vi "Convert to scripting configuration.vi"(7 "GObj Array in":refnum<vi>[](array[refnum]), 8 "error in (no error)":errorcluster, 11 "Multiple Assert Configuration":T1[](array[typedef])) -> (0 "error out":errorcluster, 3 "Array":T4[](array[typedef]), 5 "GObj Array out":refnum<vi>[](array[refnum]))   [LabVIEW 2016]
doc: "Converts the simplified multiple assert configuration array into the full scripting configuration"
uses:
  Assert Scripting Configuration.ctl
  <vilib>/Utility/Data Type/Type Definitions/Data Type.ctl
  Assert Build Configuration.ctl
  Core/Assert API Components/Failure Actions.ctl
  <vilib>/Utility/Data Type/NI_Data Type.lvlib
  Core/Assert API Components/Assert API Components.lvlib
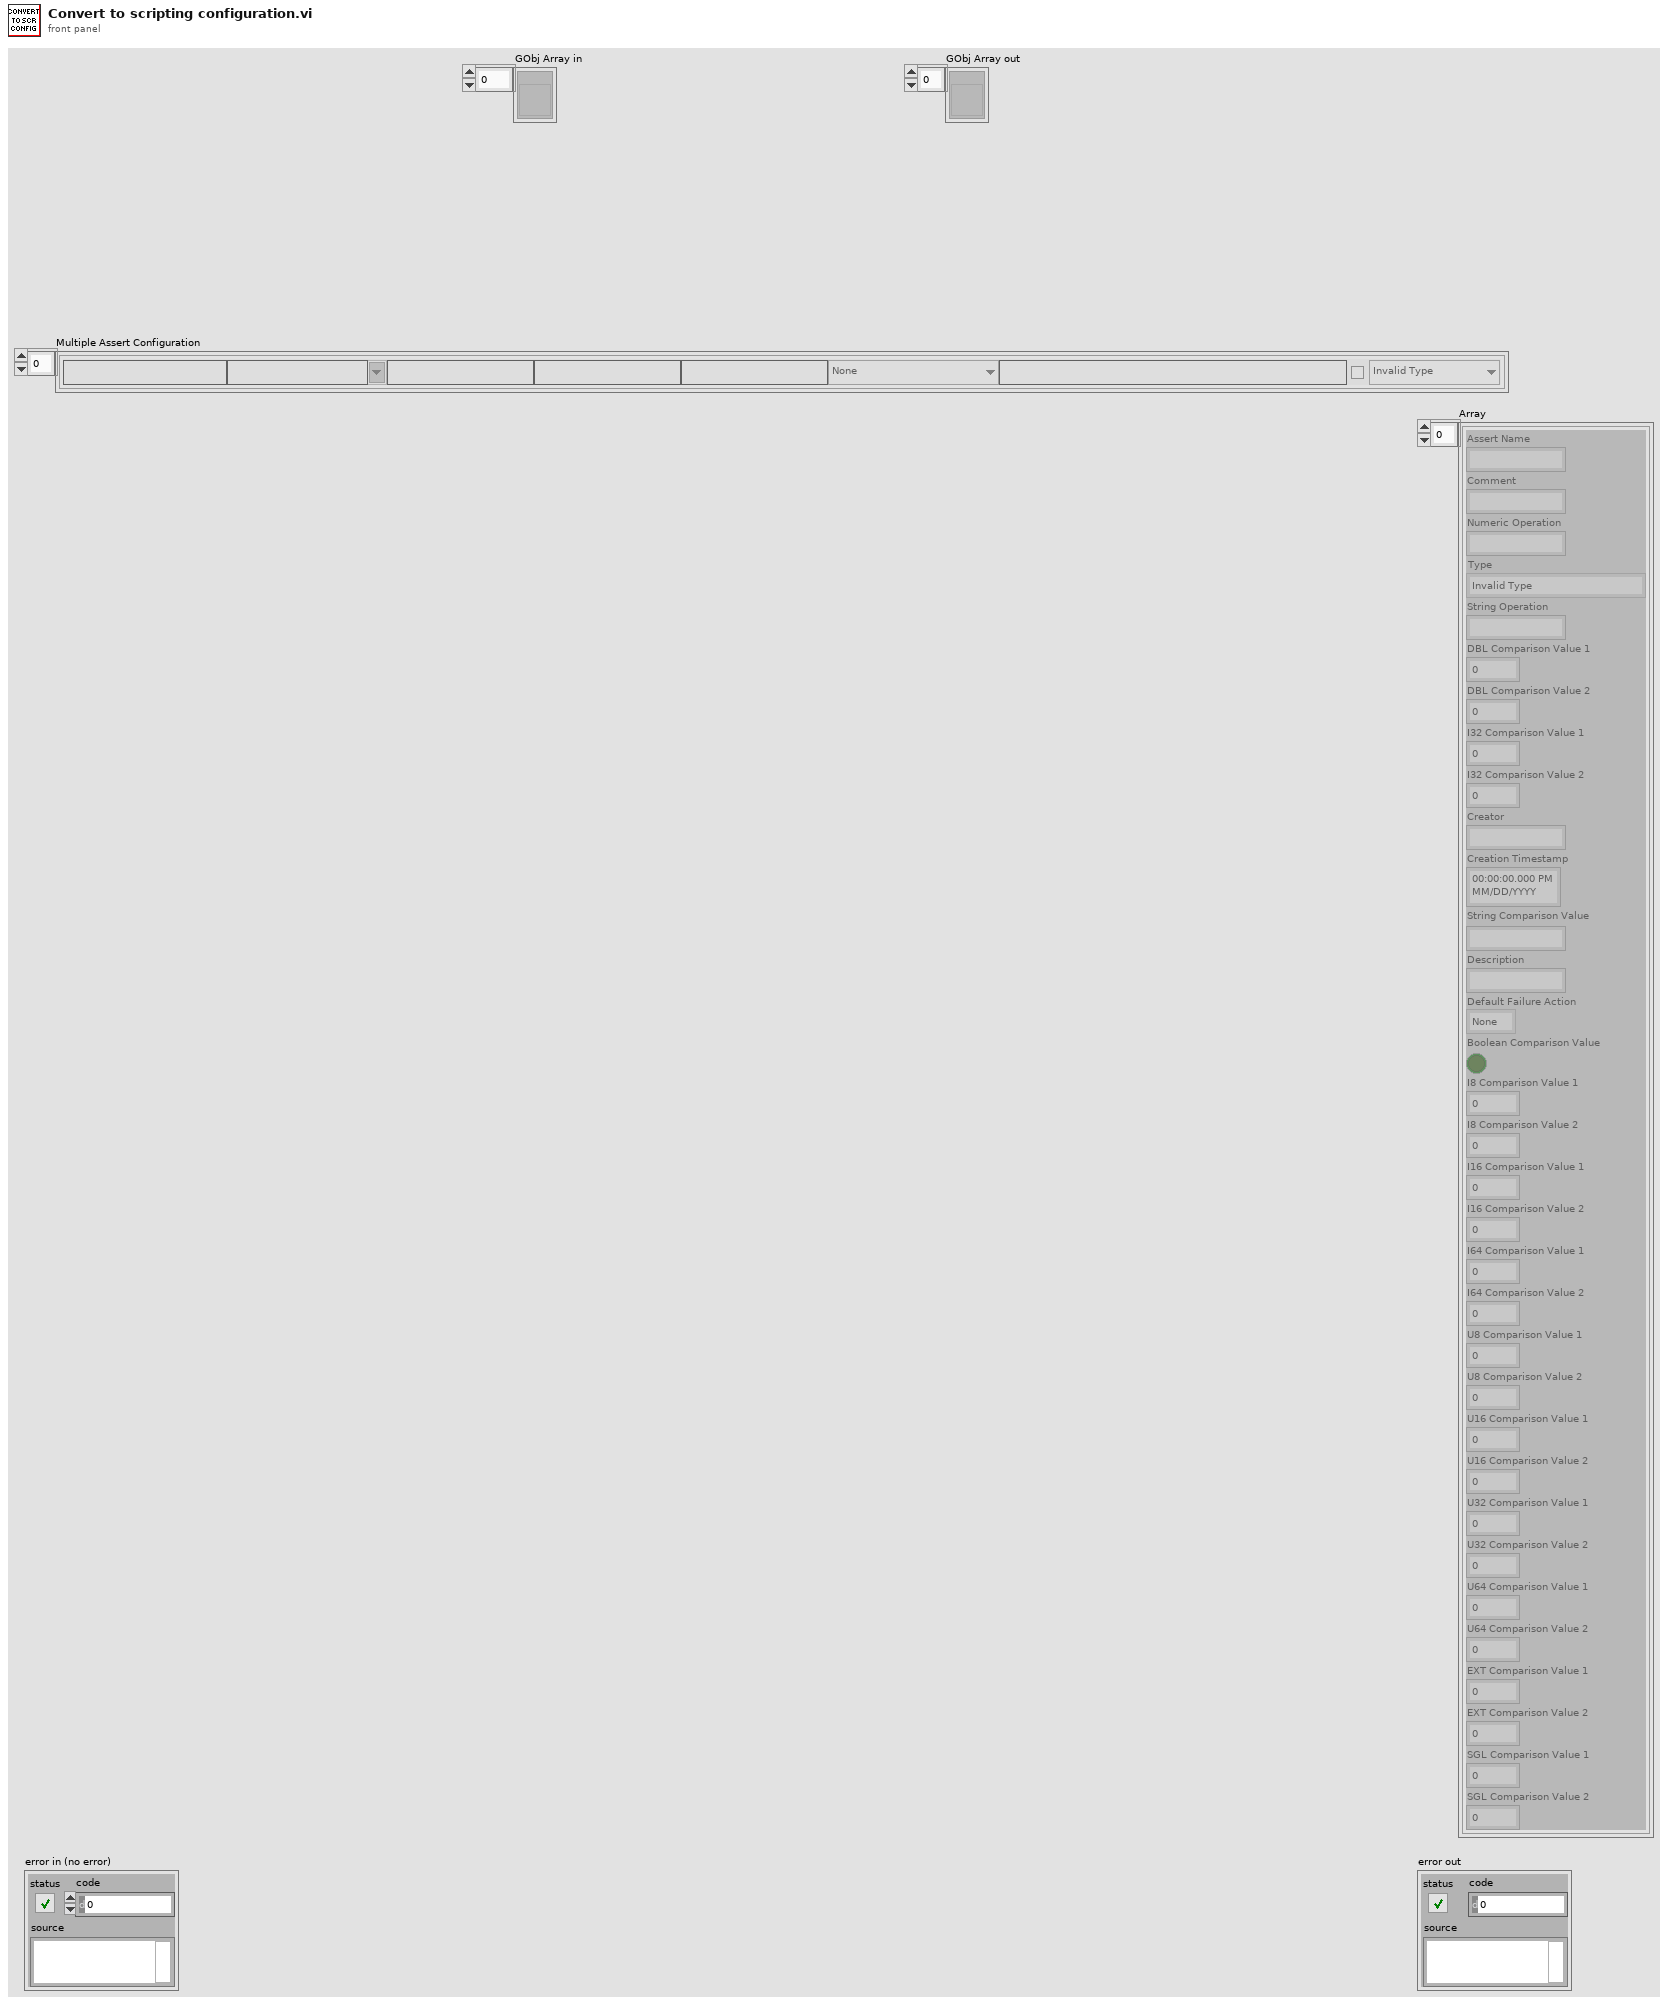
[diagram p1: front panel]
types:
  T1 = typedef "Assert Build Configuration.ctl" = cluster{"Assert Name":string, "Operation":string, "Comparison Value 1":string, "Comparison Value 2":string, "Comment":string, "Default Failure Action":T2, "Description":string, "Operation Display":string, "Active":bool, "Data Type":T3}
  T2 = typedef "Assert API Components.lvlib/Failure Actions.ctl" = enum16{"None", "Log To File", "Pause Execution", "Abort Execution"}
  T3 = typedef "NI_Data Type.lvlib/Data Type.ctl" = enum8{"Invalid Type", "Void", "I8", "I16", "I32", "I64", "U8", "U16", "U32", "U64", "Single Float", "Double Float", "Extended Float", "Single Complex", "Double Complex", "Extended Complex", "Enum U8", "Enum U16", "Enum U32", "Enum U64", "Single Float With Unit", "Double Float With Unit", "Extended Float With Unit", "Single Complex with Unit", "Double Complex with Unit", "Extended Complex with Unit", "Boolean", "String", "Path", "Picture", "Tag", "Array", "Cluster", "Variant", "LV Variant", "Waveform", "Timestamp", "Digital Waveform", "Digital Data", "ExpressData", "Refnum", "External Data", "VI", "Poly VI", "LabVIEW Class Instance", "Fixed Point"}
  T4 = typedef "Assert Scripting Configuration.ctl" = cluster{"Assert Name":string, "Comment":string, "Numeric Operation":string, "Type":T3, "String Operation":string, "DBL Comparison Value 1":dbl, "DBL Comparison Value 2":dbl, "I32 Comparison Value 1":i32, "I32 Comparison Value 2":i32, "Creator":string, "Creation Timestamp":timestamp, "String Comparison Value":string, "Description":string, "Default Failure Action":enum16{"None", "Log To File", "Pause Execution", "Abort Execution"}, "Boolean Comparison Value":bool, "I8 Comparison Value 1":i8, "I8 Comparison Value 2":i8, "I16 Comparison Value 1":i16, "I16 Comparison Value 2":i16, "I64 Comparison Value 1":i64, "I64 Comparison Value 2":i64, "U8 Comparison Value 1":u8, "U8 Comparison Value 2":u8, "U16 Comparison Value 1":u16, "U16 Comparison Value 2":u16, "U32 Comparison Value 1":u32, "U32 Comparison Value 2":u32, "U64 Comparison Value 1":u64, "U64 Comparison Value 2":u64, "EXT Comparison Value 1":ext, "EXT Comparison Value 2":ext, "SGL Comparison Value 1":sgl, "SGL Comparison Value 2":sgl}
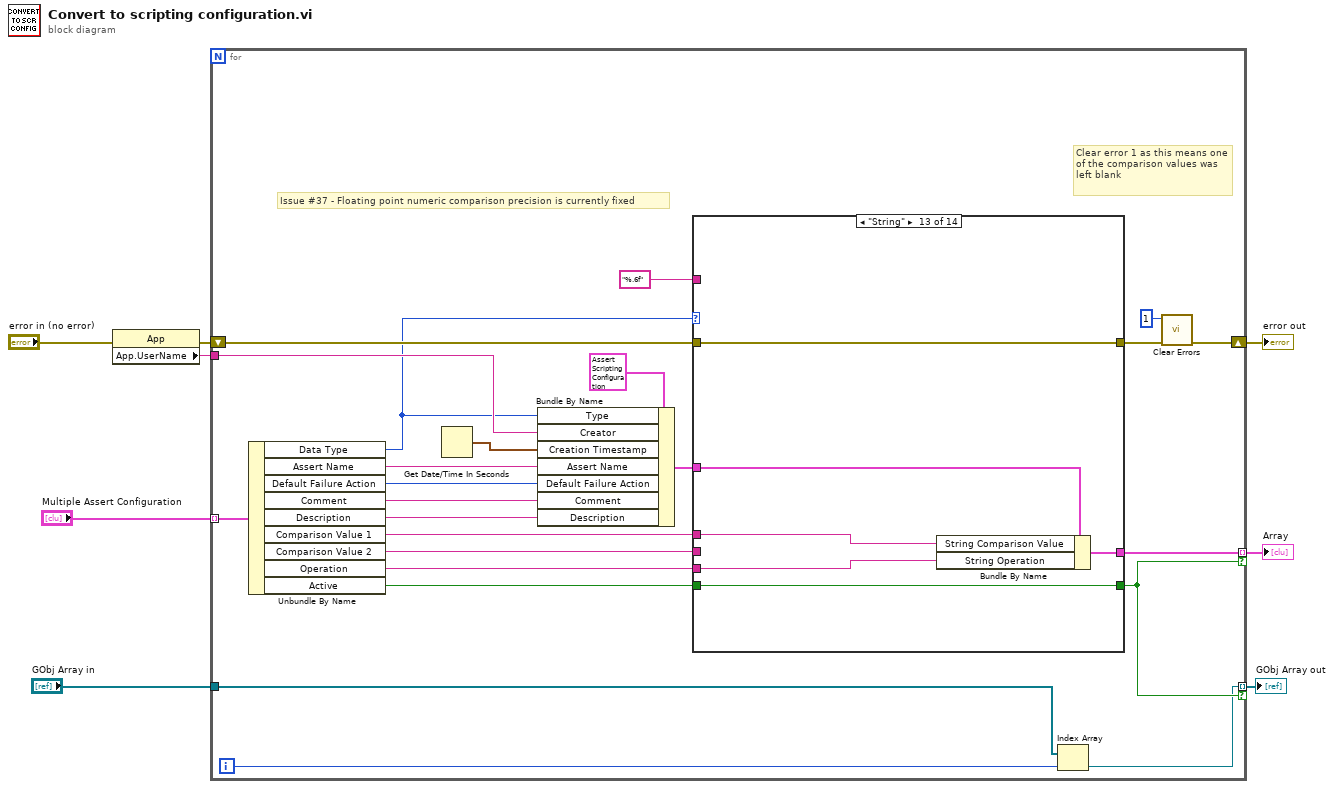
[diagram p0: block diagram]
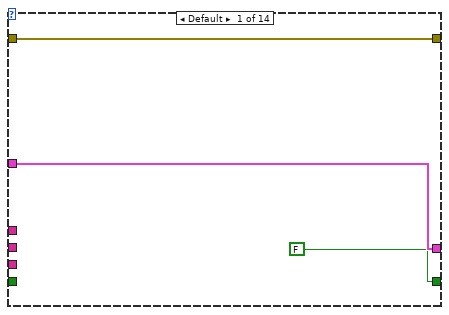
[diagram p2: hidden frame]
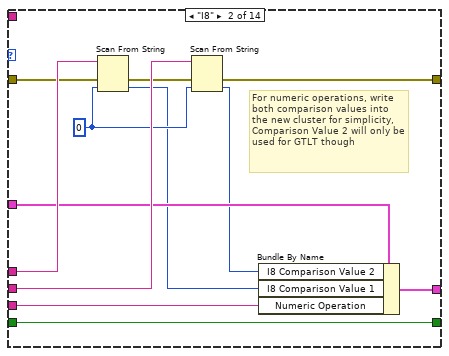
[diagram p3: hidden frame]
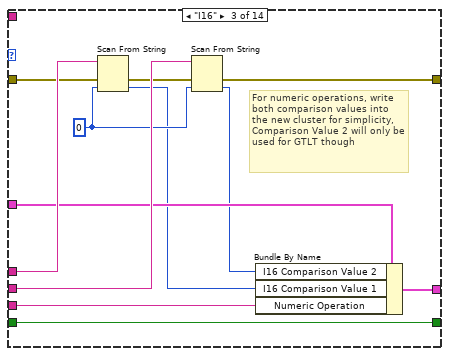
[diagram p4: hidden frame]
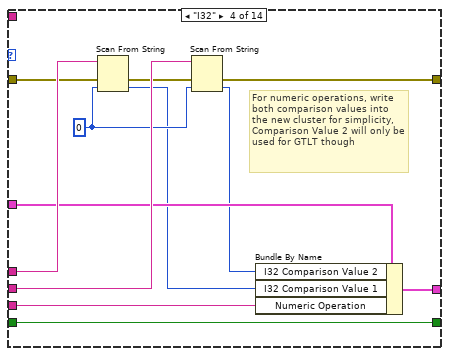
[diagram p5: hidden frame]
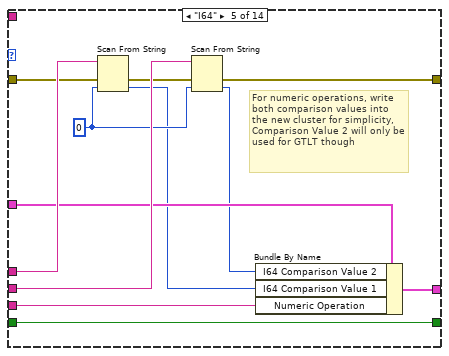
[diagram p6: hidden frame]
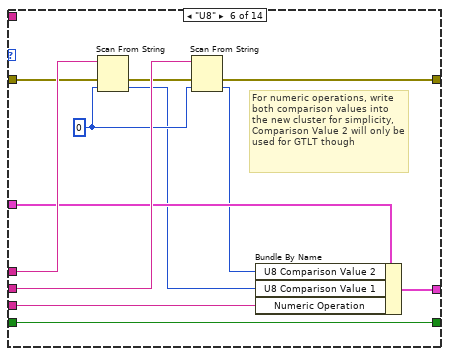
[diagram p7: hidden frame]
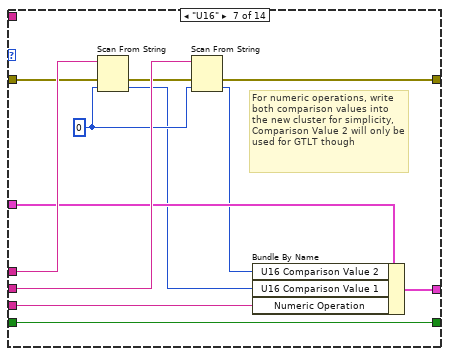
[diagram p8: hidden frame]
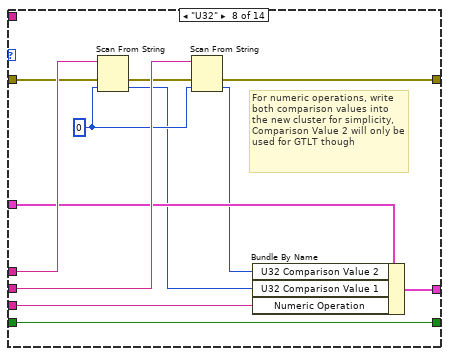
[diagram p9: hidden frame]
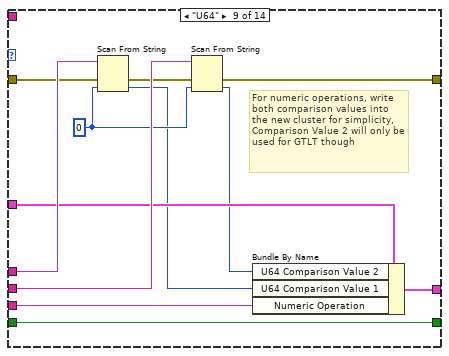
[diagram p10: hidden frame]
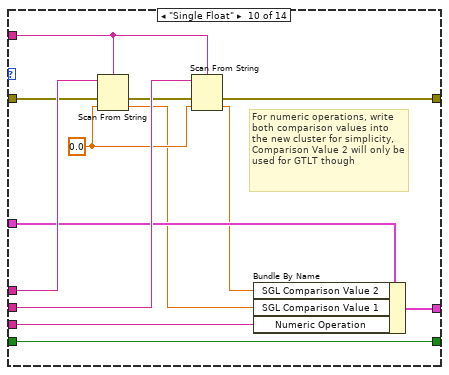
[diagram p11: hidden frame]
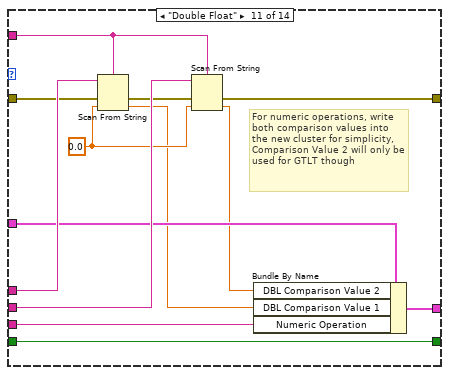
[diagram p12: hidden frame]
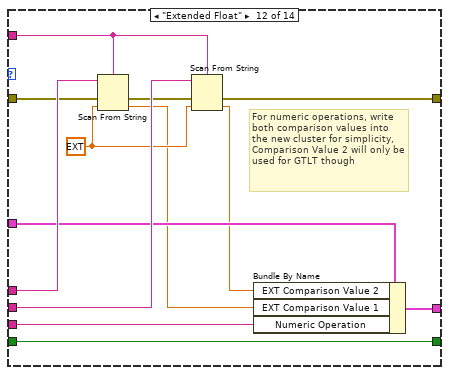
[diagram p13: hidden frame]
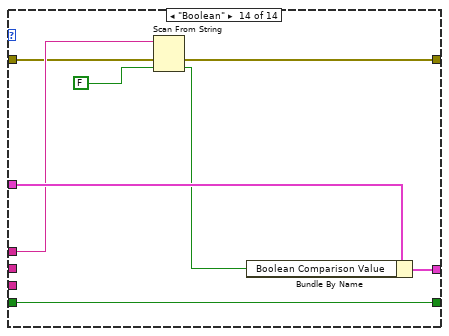
[diagram p14: hidden frame]
diagram:
  n1 = property class="App"(error in="error in (no error)") -> (error out=w5:errorcluster, "App.UserName"=w6:string)  [unwired: 1 in, 1 out]
  n2 = for {
    tunnel: "Multiple Assert Configuration" -> [w32] mode=indexing
    tunnel: w6 -> [w26]
    tunnel: [w23] -> w3 mode=indexing if=w12
    shift-right: [w15] -> w4
    shift-left: w5 -> [w19]
    tunnel: "GObj Array in" -> [w11]
    tunnel: [w9] -> w1 mode=indexing if=w12
    i -> [w10]
    # "Issue #37 - Floating point numeric comparison precision is currently fixed"
    # "Clear error 1 as this means one of the comparison values was left blank"
    n3 = Unbundle By Name(w32) -> ("Data Type"=w16:T3, "Assert Name"=w31:string, "Default Failure Action"=w30:T2, "Comment"=w29:string, "Description"=w28:string, "Comparison Value 1"=w20:string, "Comparison Value 2"=w21:string, "Operation"=w22:string, "Active"=w24:bool)
    n4 = Get Date/Time In Seconds() -> (seconds since 1Jan1904=w27:timestamp)
    n5 = Bundle By Name(cluster=T4 {"Assert Name"="", "Comment"="", "Numeric Operation"="", "Type"=enum."Double Float", "String Operation"="", "DBL Comparison Value 1"=0.0, "DBL Comparison Value 2"=0.0, "I32 Comparison Value 1"=0, "I32 Comparison Value 2"=0, "Creator"="", "Creation Timestamp"=timestamp(0 s since 1904-01-01), "String Comparison Value"="", "Description"="", "Default Failure Action"=enum."None", "Boolean Comparison Value"=FALSE, "I8 Comparison Value 1"=0, "I8 Comparison Value 2"=0, "I16 Comparison Value 1"=0, "I16 Comparison Value 2"=0, "I64 Comparison Value 1"=0, "I64 Comparison Value 2"=0, "U8 Comparison Value 1"=0, "U8 Comparison Value 2"=0, "U16 Comparison Value 1"=0, "U16 Comparison Value 2"=0, "U32 Comparison Value 1"=0, "U32 Comparison Value 2"=0, "U64 Comparison Value 1"=0, "U64 Comparison Value 2"=0, "EXT Comparison Value 1"=0.0, "EXT Comparison Value 2"=0.0, "SGL Comparison Value 1"=0.0, "SGL Comparison Value 2"=0.0} ("Assert Scripting Configuration"), "Type"=w16, "Creator"=w26, "Creation Timestamp"=w27, "Assert Name"=w31, "Default Failure Action"=w30, "Comment"=w29, "Description"=w28) -> (w25:T4)
    n6 = case shown="\"String\"" w16 {
      tunnel: w25 -> [w35 w44 w56 w68 w80 w92 w104 w116 w128 w141 w154 w167 w175 w183]
      tunnel: w24 -> [_ w45 w57 w69 w81 w93 w105 w117 w129 w142 w155 w168 w176 w184]
      tunnel: [w35 w42 w54 w66 w78 w90 w102 w114 w126 w139 w152 w165 w173 w182] -> w23
      tunnel: [FALSE w45 w57 w69 w81 w93 w105 w117 w129 w142 w155 w168 w176 w184] -> w12
      tunnel: w22 -> [_ w38 w50 w62 w74 w86 w98 w110 w122 w135 w148 w161 w172 _]
      tunnel: w21 -> [_ w47 w59 w71 w83 w95 w107 w119 w131 w144 w157 w170 _ _]
      tunnel: w20 -> [_ w46 w58 w70 w82 w94 w106 w118 w130 w143 w156 w169 w171 w181]
      tunnel: w19 -> [w33 w43 w55 w67 w79 w91 w103 w115 w127 w140 w153 w166 w174 w178]
      tunnel: [w33 w41 w53 w65 w77 w89 w101 w113 w125 w138 w151 w164 w174 w177] -> w18
      tunnel: "%.6f" ("format string") -> [_ _ _ _ _ _ _ _ _ w132 w145 w158 _ _]
      frame Default {
      }
      frame "I8" {
        w39 = i8 0
        # "For numeric operations, write both comparison values into the new cluster for simplicity, Comparison Value 2 will only be used for GTLT though"
        n7 = Scan From String(input string=w46, error in=w43, default 1=w39) -> (error out=w40:errorcluster, output 1=w36:i8)  [unwired: 2 in, 2 out]
        n8 = Scan From String(input string=w47, error in=w40, default 1=w39) -> (error out=w41:errorcluster, output 1=w37:i8)  [unwired: 2 in, 2 out]
        n9 = Bundle By Name(cluster=w44, "I8 Comparison Value 2"=w37, "I8 Comparison Value 1"=w36, "Numeric Operation"=w38) -> (w42:T4)
      }
      frame "I16" {
        w51 = i16 0
        # "For numeric operations, write both comparison values into the new cluster for simplicity, Comparison Value 2 will only be used for GTLT though"
        n10 = Scan From String(input string=w58, error in=w55, default 1=w51) -> (error out=w52:errorcluster, output 1=w48:i16)  [unwired: 2 in, 2 out]
        n11 = Scan From String(input string=w59, error in=w52, default 1=w51) -> (error out=w53:errorcluster, output 1=w49:i16)  [unwired: 2 in, 2 out]
        n12 = Bundle By Name(cluster=w56, "I16 Comparison Value 2"=w49, "I16 Comparison Value 1"=w48, "Numeric Operation"=w50) -> (w54:T4)
      }
      frame "I32" {
        w63 = 0
        # "For numeric operations, write both comparison values into the new cluster for simplicity, Comparison Value 2 will only be used for GTLT though"
        n13 = Scan From String(input string=w70, error in=w67, default 1=w63) -> (error out=w64:errorcluster, output 1=w60:i32)  [unwired: 2 in, 2 out]
        n14 = Scan From String(input string=w71, error in=w64, default 1=w63) -> (error out=w65:errorcluster, output 1=w61:i32)  [unwired: 2 in, 2 out]
        n15 = Bundle By Name(cluster=w68, "I32 Comparison Value 2"=w61, "I32 Comparison Value 1"=w60, "Numeric Operation"=w62) -> (w66:T4)
      }
      frame "I64" {
        w75 = i64 0
        # "For numeric operations, write both comparison values into the new cluster for simplicity, Comparison Value 2 will only be used for GTLT though"
        n16 = Scan From String(input string=w82, error in=w79, default 1=w75) -> (error out=w76:errorcluster, output 1=w72:i64)  [unwired: 2 in, 2 out]
        n17 = Scan From String(input string=w83, error in=w76, default 1=w75) -> (error out=w77:errorcluster, output 1=w73:i64)  [unwired: 2 in, 2 out]
        n18 = Bundle By Name(cluster=w80, "I64 Comparison Value 2"=w73, "I64 Comparison Value 1"=w72, "Numeric Operation"=w74) -> (w78:T4)
      }
      frame "U8" {
        w87 = u8 0
        # "For numeric operations, write both comparison values into the new cluster for simplicity, Comparison Value 2 will only be used for GTLT though"
        n19 = Scan From String(input string=w94, error in=w91, default 1=w87) -> (error out=w88:errorcluster, output 1=w84:u8)  [unwired: 2 in, 2 out]
        n20 = Scan From String(input string=w95, error in=w88, default 1=w87) -> (error out=w89:errorcluster, output 1=w85:u8)  [unwired: 2 in, 2 out]
        n21 = Bundle By Name(cluster=w92, "U8 Comparison Value 2"=w85, "U8 Comparison Value 1"=w84, "Numeric Operation"=w86) -> (w90:T4)
      }
      frame "U16" {
        w99 = u16 0
        # "For numeric operations, write both comparison values into the new cluster for simplicity, Comparison Value 2 will only be used for GTLT though"
        n22 = Scan From String(input string=w106, error in=w103, default 1=w99) -> (error out=w100:errorcluster, output 1=w96:u16)  [unwired: 2 in, 2 out]
        n23 = Scan From String(input string=w107, error in=w100, default 1=w99) -> (error out=w101:errorcluster, output 1=w97:u16)  [unwired: 2 in, 2 out]
        n24 = Bundle By Name(cluster=w104, "U16 Comparison Value 2"=w97, "U16 Comparison Value 1"=w96, "Numeric Operation"=w98) -> (w102:T4)
      }
      frame "U32" {
        w111 = u32 0
        # "For numeric operations, write both comparison values into the new cluster for simplicity, Comparison Value 2 will only be used for GTLT though"
        n25 = Scan From String(input string=w118, error in=w115, default 1=w111) -> (error out=w112:errorcluster, output 1=w108:u32)  [unwired: 2 in, 2 out]
        n26 = Scan From String(input string=w119, error in=w112, default 1=w111) -> (error out=w113:errorcluster, output 1=w109:u32)  [unwired: 2 in, 2 out]
        n27 = Bundle By Name(cluster=w116, "U32 Comparison Value 2"=w109, "U32 Comparison Value 1"=w108, "Numeric Operation"=w110) -> (w114:T4)
      }
      frame "U64" {
        w123 = u64 0
        # "For numeric operations, write both comparison values into the new cluster for simplicity, Comparison Value 2 will only be used for GTLT though"
        n28 = Scan From String(input string=w130, error in=w127, default 1=w123) -> (error out=w124:errorcluster, output 1=w120:u64)  [unwired: 2 in, 2 out]
        n29 = Scan From String(input string=w131, error in=w124, default 1=w123) -> (error out=w125:errorcluster, output 1=w121:u64)  [unwired: 2 in, 2 out]
        n30 = Bundle By Name(cluster=w128, "U64 Comparison Value 2"=w121, "U64 Comparison Value 1"=w120, "Numeric Operation"=w122) -> (w126:T4)
      }
      frame "Single Float" {
        w136 = sgl 0.0
        # "For numeric operations, write both comparison values into the new cluster for simplicity, Comparison Value 2 will only be used for GTLT though"
        n31 = Scan From String(format string=w132, input string=w143, error in=w140, default 1=w136) -> (error out=w137:errorcluster, output 1=w133:sgl)  [unwired: 1 in, 2 out]
        n32 = Scan From String(format string=w132, input string=w144, error in=w137, default 1=w136) -> (error out=w138:errorcluster, output 1=w134:sgl)  [unwired: 1 in, 2 out]
        n33 = Bundle By Name(cluster=w141, "SGL Comparison Value 2"=w134, "SGL Comparison Value 1"=w133, "Numeric Operation"=w135) -> (w139:T4)
      }
      frame "Double Float" {
        w149 = 0.0
        # "For numeric operations, write both comparison values into the new cluster for simplicity, Comparison Value 2 will only be used for GTLT though"
        n34 = Scan From String(format string=w145, input string=w156, error in=w153, default 1=w149) -> (error out=w150:errorcluster, output 1=w146:dbl)  [unwired: 1 in, 2 out]
        n35 = Scan From String(format string=w145, input string=w157, error in=w150, default 1=w149) -> (error out=w151:errorcluster, output 1=w147:dbl)  [unwired: 1 in, 2 out]
        n36 = Bundle By Name(cluster=w154, "DBL Comparison Value 2"=w147, "DBL Comparison Value 1"=w146, "Numeric Operation"=w148) -> (w152:T4)
      }
      frame "Extended Float" {
        w162 = ext 0.0
        # "For numeric operations, write both comparison values into the new cluster for simplicity, Comparison Value 2 will only be used for GTLT though"
        n37 = Scan From String(format string=w158, input string=w169, error in=w166, default 1=w162) -> (error out=w163:errorcluster, output 1=w159:ext)  [unwired: 1 in, 2 out]
        n38 = Scan From String(format string=w158, input string=w170, error in=w163, default 1=w162) -> (error out=w164:errorcluster, output 1=w160:ext)  [unwired: 1 in, 2 out]
        n39 = Bundle By Name(cluster=w167, "EXT Comparison Value 2"=w160, "EXT Comparison Value 1"=w159, "Numeric Operation"=w161) -> (w165:T4)
      }
      frame "String" {
        n40 = Bundle By Name(cluster=w175, "String Comparison Value"=w171, "String Operation"=w172) -> (w173:T4)
      }
      frame "Boolean" {
        n41 = Scan From String(input string=w181, error in=w178, default 1=FALSE) -> (error out=w177:errorcluster, output 1=w180:bool)  [unwired: 2 in, 2 out]
        n42 = Bundle By Name(cluster=w183, "Boolean Comparison Value"=w180) -> (w182:T4)
      }
    }
    n43 = Index Array(array=w11, index=w10) -> (element=w9:refnum<vi>)
    n44 = call <vilib>:"Clear Errors.vi"("error in (no error)"=w18, "specific error code to clear (0: all)"=1) -> ("error out"=w15:errorcluster)  [unwired: 4 in, 1 out]
  }
  "Array" <- w3
  "error out" <- w4
  "GObj Array out" <- w1
